vi "Configure Device.vi"(8 "error in":errorcluster, 11 "IMAQdx Base Configure Strategy in":refnum<class "IMAQdx Base Configure Strategy.lvclass">) -> (0 "error out":errorcluster, 3 "IMAQdx Base Configure Strategy out":refnum<class "IMAQdx Base Configure Strategy.lvclass">)   [LabVIEW 2024, in "IMAQdx Base Configure Strategy.lvclass"]
uses:
  IMAQdx Base Configure Strategy.lvclass
  IMAQdx Base Configure Strategy.lvclass/IMAQdx Base Configure Strategy.ctl
  Source/Interfaces/IConfiguration/IConfiguration.lvclass
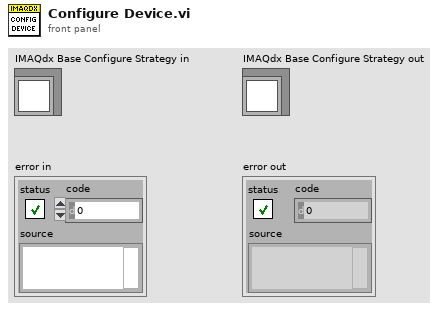
[diagram p1: front panel]
types:
  T1 = typedef "IMAQdx.ctl" = refnum<k21>
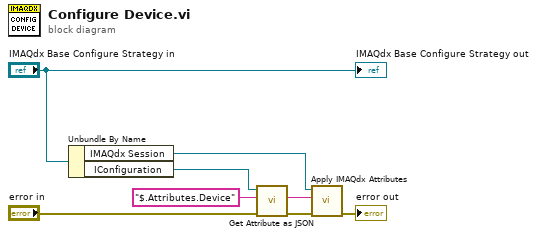
[diagram p0: block diagram]
diagram:
  n1 = Unbundle By Name("IMAQdx Base Configure Strategy in") -> ("IMAQdx Session"=w3:T1, "IConfiguration"=w1:refnum<class "IConfiguration.lvclass">)
  n2 = call-dynamic "Get Attribute as JSON.vi"("error in"="error in", "Attribute"="$.Attributes.Device", "IConfiguration in"=w1) -> ("error out"=w5:errorcluster, "<JSON>"=w2:string)  [unwired: 6 in, 1 out]
  n3 = call "Apply IMAQdx Attributes.vi"("error in"=w5, "<JSON>"=w2, "IMAQdx Session in"=w3) -> ("error out"=→"error out":errorcluster)  [unwired: 7 in, 1 out]
  "IMAQdx Base Configure Strategy out" <- "IMAQdx Base Configure Strategy in"
